vi "TestXNEt.vi"() -> ()   [LabVIEW 2021]
uses:
  <vilib>/FPGAPlugInAG/cRIO-9068/niLvFpga_Open_cRIO-9068.vi
  <vilib>/FPGAPlugInAG/cRIO-9068/niLvFpga_Run_cRIO-9068.vi
  <vilib>/rvi/interface/nirviOpenFPGA/nirviOpenFPGA.xnode
  FPGA Bitfiles/pv-emulators_FPGATarget_emptyFPGA_z5uule7UYNw.lvbitx
  <vilib>/rvi/interface/nirviMethod/nirviMethod.xnode
  <resource>/objmgr/xnet.rc
panel:
  out "FPGA VI Reference Out":refnum<k20>
  out "error out":errorcluster
  out "Interfaces (Ethernet)":refnum<k21>[](array[refnum])
  out "Interfaces (CAN)":refnum<k21>[](array[refnum])
  out "Devices":refnum<k21>[](array[refnum])
  in  "stop":bool
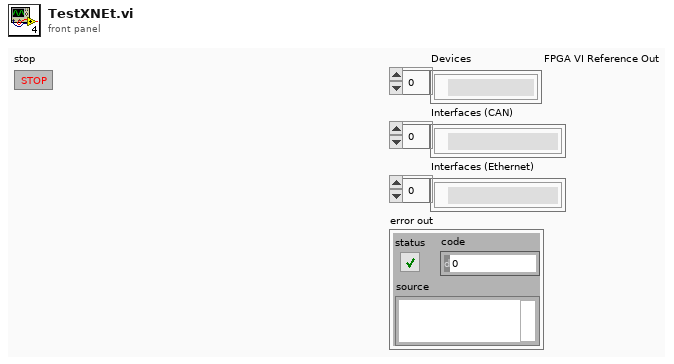
[diagram p1: front panel]
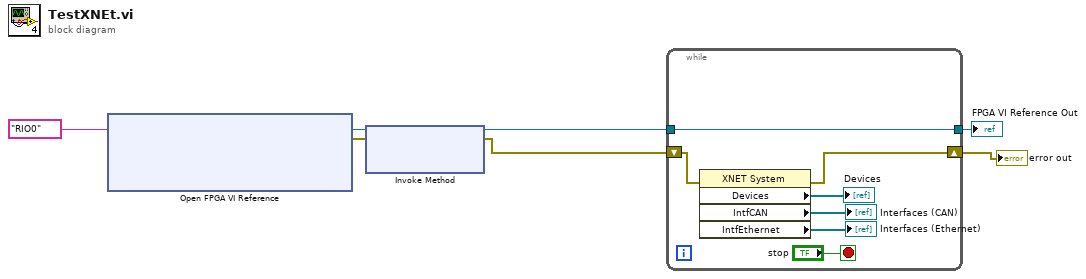
[diagram p0: block diagram]
diagram:
  n1 = xnode "Open FPGA VI Reference"("resource name"=tag "RIO0") -> ("FPGA VI Reference Out"=w3:refnum<k20>, "error out"=w7:errorcluster)  [unwired: 1 in]
  n2 = xnode "Invoke Method"("FPGA VI Reference In"=w3, "error in"=w7) -> ("FPGA VI Reference Out"=w2:refnum<k20>, "error out"=w5:errorcluster)  [unwired: 1 in]
  n3 = while {
    tunnel: w2 -> [w8]
    shift-right: [w9] -> w4
    shift-left: w5 -> [w10]
    tunnel: [w8] -> w1
    stop <- "stop" stop-if-true
    n4 = property class="XNET System"(error in=w10) -> (error out=w9:errorcluster, "Devices"=→"Devices":refnum<k21>[], "IntfCAN"=→"Interfaces (CAN)":refnum<k21>[], "IntfEthernet"=→"Interfaces (Ethernet)":refnum<k21>[])  [unwired: 1 in, 1 out]
  }
  "error out" <- w4
  "FPGA VI Reference Out" <- w1
